vi "CURVA.vi"() -> ()   [LabVIEW 2018]
uses:
  <vilib>/Instr/_visa.llb/VISA Configure Serial Port (Instr).vi
panel:
  out "CURVA FRECUENCIA RESPIRATORIA":dbl(graph)
  in  "Puerto COM":refnum<visa-resource-name>
  # "MONITOR DE FRECUENCIA RESPIRATORIA"
  # "PROYECTO DE CÁTEDRA\nBIOINTRUMENTACIÓN 2019"
  # "La apnea se puede denominar como una patología respiratoria que se lleva a cabo cuando quien lo \npadece, tiende a presentar interrupciones en su respiración. Este tipo de dolencias se ven más frecuentemente durante el sueño es por ello que es conocida como apnea del sueño; siendo ésta más \ncomún de lo que se podría imaginar, ya que afecta \na más de 3 hombres de cada 10 y a casi 1 mujer de cada 5."
  # "La apnea del sueño puede hacer peligrar la vida puesto que se ve asociada a un latido irregular del corazón, alta presión sanguínea o a un ataque cardíaco. Ésta produce por la relajación de los músculos de la parte superior de la garganta, provocando que estos tejidos se cierren bloqueando la vía respiratoria."
  # "Creado por:  Argueta Argueta, Kevin Josué (AA170194), Fuentes Escolero, Edwin Antonio (FE170732), Mendoza Orellana, Adriana María (MO170241)"
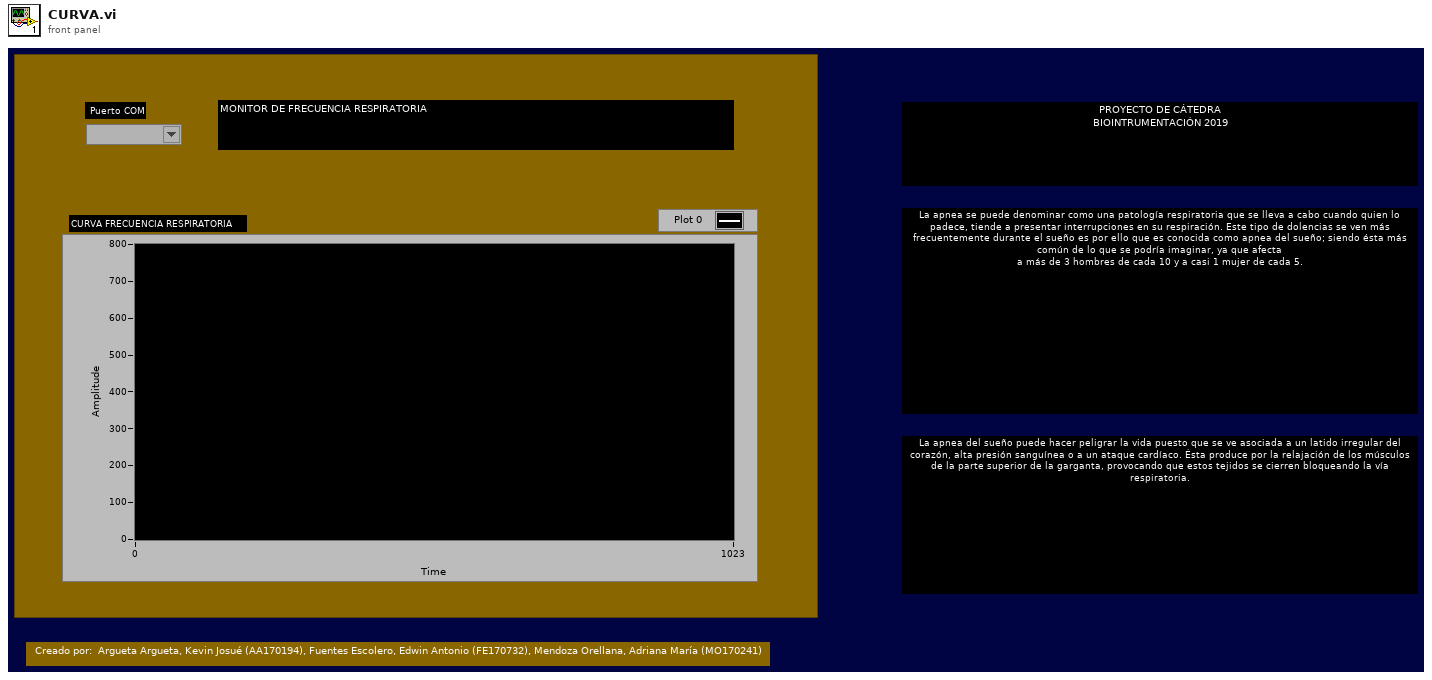
[diagram p1: front panel]
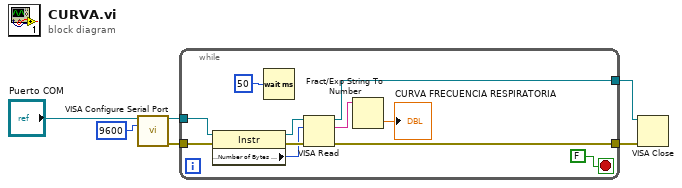
[diagram p0: block diagram]
diagram:
  n1 = call-poly "VISA Configure Serial Port"("VISA resource name"="Puerto COM", "baud rate (9600)"=u32 9600) -> ("VISA resource name out"=w6:refnum<visa-resource-name>, "error out"=w5:errorcluster)  [unwired: 12 in]
  n2 = while {
    tunnel: w6 -> [w17]
    tunnel: w5 -> [w16]
    tunnel: [w14] -> w4
    tunnel: [w13] -> w3
    stop <- FALSE stop-if-true
    n3 = property class="Instr"(reference=w17, error in=w16) -> (reference out=w15:refnum<visa-resource-name>, error out=w12:errorcluster, "Serial Settings:Number of Bytes at Serial Port"=w11:u32)
    n4 = Wait (ms)(milliseconds to wait=u32 50) -> ()  [unwired: 1 out]
    n5 = VISA Read(VISA resource name=w15, byte count=w11, error in (no error)=w12) -> (VISA resource name out=w14:refnum<visa-resource-name>, read buffer=w10:string, error out=w13:errorcluster)  [unwired: 1 out]
    n6 = Fract/Exp String To Number(string=w10) -> (number=→"CURVA FRECUENCIA RESPIRATORIA":dbl)  [unwired: 3 in, 1 out]
  }
  n7 = VISA Close(VISA resource name=w4, error in (no error)=w3) -> ()  [unwired: 1 out]
